vi "Set Hash.vi"(8 "error in (no error)":errorcluster, 10 "Hash":refnum<class "Hash.lvclass">, 11 "HMAC in":refnum<class "HMAC.lvclass">) -> (0 "error out":errorcluster, 3 "HMAC out":refnum<class "HMAC.lvclass">)   [LabVIEW 2020, in "Crypto.lvlib" / "HMAC.lvclass"]
uses:
  HMAC.lvclass
  Hash/Hash.lvclass
  HMAC.lvclass/HMAC.ctl
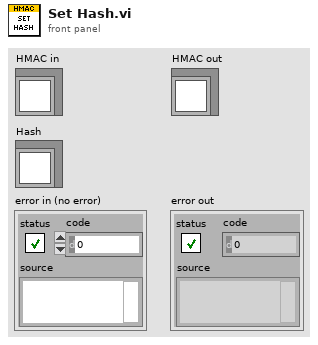
[diagram p1: front panel]
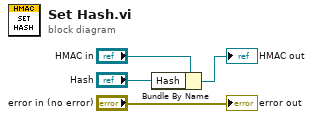
[diagram p0: block diagram]
diagram:
  n1 = Bundle By Name(cluster="HMAC in", "Hash"="Hash") -> (→"HMAC out":refnum<class "HMAC.lvclass">)
  "error out" <- "error in (no error)"
